vi "ex_sample data.vi"() -> (0 "Signals":waveform(dbl)(graph))   [LabVIEW 2020]
doc: "Sample sinewave used by several of the measurement Express VI property pages."
uses:
  <vilib>/measure/NI_MABase.lvlib
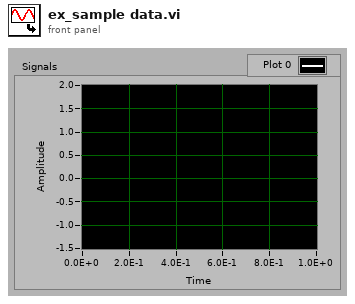
[diagram p1: front panel]
types:
  T1 = cluster{"frequency":dbl, "amplitude":dbl, "phase":dbl}[]
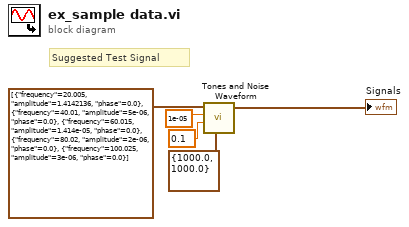
[diagram p0: block diagram]
diagram:
  # "Suggested Test Signal"
  n1 = call <vilib>:"Tones and Noise Waveform.vi"("sampling info"=cluster{"Fs":dbl, "#s":dbl} {"Fs"=1000.0, "#s"=1000.0}, "offset"=0.1, "noise (rms)"=1e-05, "tones"=T1 [{"frequency"=20.005, "amplitude"=1.4142136, "phase"=0.0}, {"frequency"=40.01, "amplitude"=5e-06, "phase"=0.0}, {"frequency"=60.015, "amplitude"=1.414e-05, "phase"=0.0}, {"frequency"=80.02, "amplitude"=2e-06, "phase"=0.0}, {"frequency"=100.025, "amplitude"=3e-06, "phase"=0.0}]) -> ("signal out"=→"Signals":waveform(dbl))  [unwired: 6 in, 1 out]
